vi "Exemple.vi"() -> ()   [LabVIEW 2020]
uses:
  <vilib>/regexp/Match Regular Expression.xnode
panel:
  out "après la correspondance":string
  out "toute l'expression":string
  out "avant la correspondance":string
  # "00077571_A|1|PCS||050666|"
  # "[\\w]+_[A-Z]\\|[0-9]\\|PCS\\|\\|[0-9]+\\|"
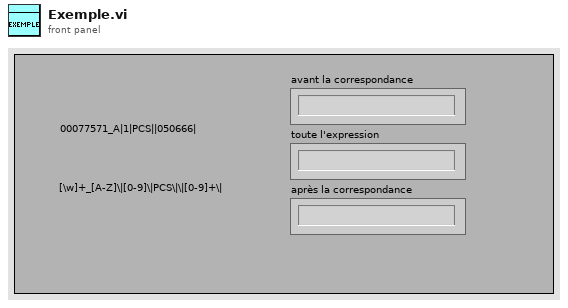
[diagram p1: front panel]
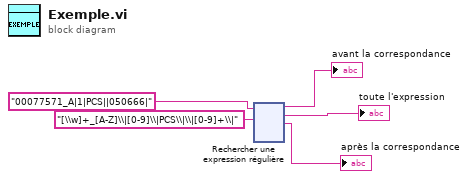
[diagram p0: block diagram]
diagram:
  n1 = xnode "Rechercher une expression régulière"("chaîne en entrée"="00077571_A|1|PCS||050666|", "expression régulière"="[\\w]+_[A-Z]\\|[0-9]\\|PCS\\|\\|[0-9]+\\|") -> ("avant la correspondance"=→"avant la correspondance":string, "toute l'expression"=→"toute l'expression":string, "après la correspondance"=→"après la correspondance":string)  [unwired: 4 in, 2 out]
